vi "file_naming_convention.vi"() -> (3 "output_filename":string)   [LabVIEW 2019]
panel:
  in  "Press When Done":bool
  in  "Select Lab Time":string(combo)
  in  "Select Course":string(combo)
  in  "Enter Group Number":string
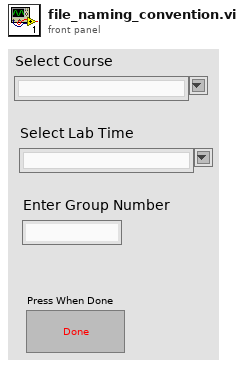
[diagram p1: front panel]
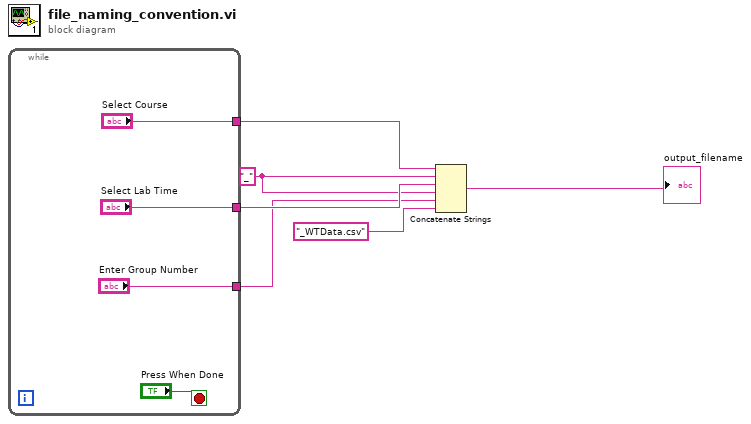
[diagram p0: block diagram]
diagram:
  w4 = "_" ("string")
  n1 = while {
    tunnel: ["Select Course"] -> w6
    tunnel: ["Select Lab Time"] -> w5
    tunnel: ["Enter Group Number"] -> w3
    stop <- "Press When Done" stop-if-true
  }
  n2 = Concatenate Strings(w6, w4, w5, w4, w3, "_WTData.csv" ("string")) -> (→"output_filename":string)
